vi "Center Window on Parent.vi"(8 "error in (no error)":errorcluster, 10 "Parent VI":refnum<vi>, 11 "VI in":refnum<vi>) -> (0 "error out":errorcluster, 3 "VI out":refnum<vi>)   [LabVIEW 2020]
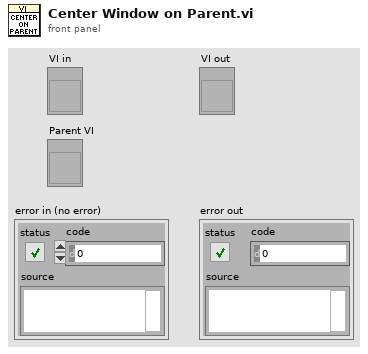
[diagram p1: front panel]
types:
  T1 = typedef "LVRectTypeDef.ctl" = cluster{"Left":i16, "Top":i16, "Right":i16, "Bottom":i16}
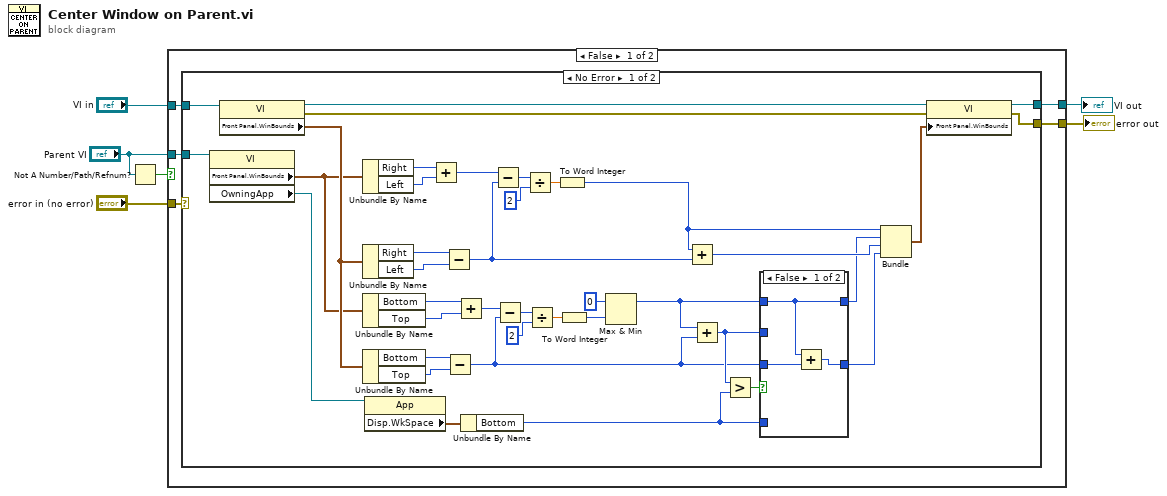
[diagram p0: block diagram]
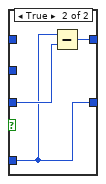
[diagram p2: hidden frame]
diagram:
  n1 = Not A Number/Path/Refnum?(number/path/refnum="Parent VI") -> (NaN/Path/Refnum?=w1:bool)
  n2 = case shown="False" w1 {
    tunnel: [w11 w58] -> w6
    tunnel: [w10 w59] -> w5
    tunnel: "error in (no error)" -> [w9 w59]
    tunnel: "VI in" -> [w8 w58]
    tunnel: "Parent VI" -> [w7 _]
    frame False {
      n3 = case shown="No Error" w9 {
        tunnel: w8 -> [w50 w57]
        tunnel: [w46 _] -> w10
        tunnel: [w47 w57] -> w11
        tunnel: w7 -> [w30 _]
        frame No Error {
          n4 = property class="VI"(reference=w30) -> ("Front Panel.WinBounds"=w24:T1, "OwningApp"=w20:refnum<vi>)  [unwired: 1 in, 2 out]
          n5 = property class="VI"(reference=w50) -> (reference out=w48:refnum<vi>, error out=w49:errorcluster, "Front Panel.WinBounds"=w32:T1)  [unwired: 1 in]
          n6 = Unbundle By Name(w24) -> ("Right"=w29:i16, "Left"=w28:i16)
          n7 = Unbundle By Name(w32) -> ("Right"=w45:i16, "Left"=w44:i16)
          n8 = Unbundle By Name(w24) -> ("Bottom"=w26:i16, "Top"=w25:i16)
          n9 = Unbundle By Name(w32) -> ("Bottom"=w43:i16, "Top"=w42:i16)
          n10 = property class="App"(reference=w20) -> ("Disp.WkSpace"=w19:T1)  [unwired: 1 in, 2 out]
          n11 = Add(x=w29, y=w28) -> (x+y=w27:i16)
          n12 = Subtract(x=w45, y=w44) -> (x-y=w34:i16)
          n13 = Subtract(x=w43, y=w42) -> (x-y=w12:i16)
          n14 = Add(x=w26, y=w25) -> (x+y=w23:i16)
          n15 = Unbundle By Name(w19) -> ("Bottom"=w17:i16)
          n16 = Subtract(x=w27, y=w34) -> (x-y=w41:i16)
          n17 = Subtract(x=w23, y=w12) -> (x-y=w38:i16)
          n18 = Divide(x=w41, y=2) -> (x/y=w39:dbl)
          n19 = Divide(x=w38, y=2) -> (x/y=w36:dbl)
          n20 = To Word Integer(number=w39) -> (16bit integer=w35:i16)
          n21 = To Word Integer(number=w36) -> (16bit integer=w22:i16)
          n22 = Max & Min(x=i16 0, y=w22) -> (max(x,y)=w15:i16)  [unwired: 1 out]
          n23 = Add(x=w35, y=w34) -> (x+y=w33:i16)
          n24 = Add(x=w15, y=w12) -> (x+y=w16:i16)
          n25 = Greater?(x=w16, y=w17) -> (0:w18:bool)
          n26 = case shown="False" w18 {
            tunnel: w17 -> [_ w54]
            tunnel: w16 -> [_ _]
            tunnel: w15 -> [w52 _]
            tunnel: [w51 w54] -> w14
            tunnel: [w52 w56] -> w13
            tunnel: w12 -> [w53 w55]
            frame False {
              n27 = Add(x=w52, y=w53) -> (x+y=w51:i16)
            }
            frame True {
              n28 = Subtract(x=w54, y=w55) -> (x-y=w56:i16)
            }
          }
          n29 = Bundle(w35, w13, w33, "Bottom"=w14) -> (w31:cluster{i16, i16, i16, "Bottom":i16})  [unwired: 1 in]
          n30 = property class="VI"(reference=w48, error in=w49, "Front Panel.WinBounds"=w31) -> (reference out=w47:refnum<vi>, error out=w46:errorcluster)
        }
        frame Error {
        }
      }
    }
    frame True {
    }
  }
  "VI out" <- w6
  "error out" <- w5
